vi "Анализ выхода за границы мишени (SubVI).vi"(5 "Ref мишени":refnum<vi>, 8 "Ref XY лазера":refnum<vi>, 9 "error in":errorcluster, 10 "Шаг перехода":string) -> (12 "Шаг перехода вых":string, 14 "вышел за рамки сверху":bool, 15 "вышел за рамки снизу":bool, 16 "вышел за рамки слева":bool, 17 "вышел за рамки справа":bool, 19 "error out":errorcluster)   [LabVIEW 2013]
doc: "Анализ нахождения лазера внутри мишени..."
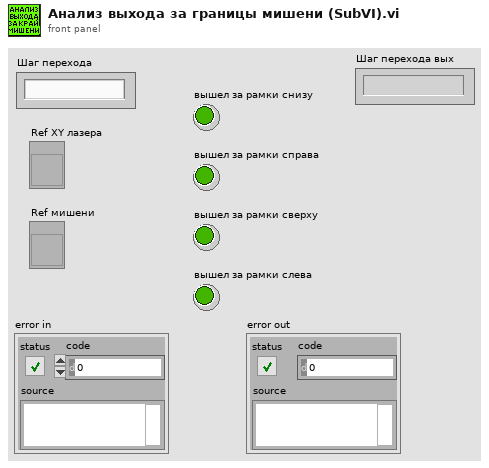
[diagram p1: front panel]
types:
  T1 = typedef "LVPositionTypeDef.ctl" = cluster{"Left":i32, "Top":i32}
  T2 = typedef "LVBoundsTypeDef.ctl" = cluster{"Width":u32, "Height":u32}
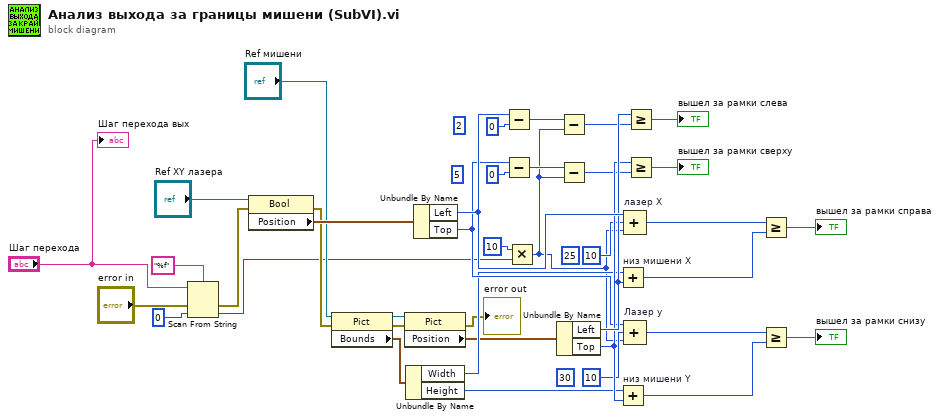
[diagram p0: block diagram]
diagram:
  (unwired) 30 ("y")
  (unwired) 25 ("y")
  (unwired) 5 ("y")
  (unwired) 2 ("y")
  n1 = Scan From String(format string="%f", input string="Шаг перехода", error in="error in", default 1=u8 0 ("element")) -> (error out=w8:errorcluster, output 1=w13:u8)  [unwired: 1 in, 2 out]
  n2 = property on="Property Node" class="Bool"(reference="Ref XY лазера", error in=w8) -> (error out=w16:errorcluster, "Position"=w20:T1)  [unwired: 1 out]
  n3 = property on="Property Node" class="Pict"(reference="Ref мишени", error in=w16) -> (reference out=w7:refnum<vi>, error out=w15:errorcluster, "Bounds"=w23:T2)
  n4 = property on="Property Node" class="Pict"(reference=w7, error in=w15) -> (error out=→"error out":errorcluster, "Position"=w19:T1)  [unwired: 1 out]
  n5 = Unbundle By Name(w23) -> ("Width"=w25:u32, "Height"=w24:u32)
  n6 = Unbundle By Name(w20) -> ("Left"=w36:i32, "Top"=w31:i32)
  n7 = Subtract(x=w36, y=0) -> (x-y=w5:i32)
  n8 = Subtract(x=w31, y=0) -> (x-y=w3:i32)
  n9 = Multiply(x=u8 10 ("element"), y=w13) -> (x*y=w2:u8)
  n10 = Unbundle By Name(w19) -> ("Left"=w33:i32, "Top"=w32:i32)
  n11 = Subtract(x=w5, y=w2) -> (x-y=w4:i32)
  n12 = Subtract(x=w3, y=w2) -> (x-y=w1:i32)
  n13 = Add "низ мишени X"(x=w25, y=w33) -> (x+y=w26:u32)
  n14 = Add "низ мишени Y"(x=w24, y=w32) -> (x+y=w39:u32)
  n15 = Compound Arithmetic op=ADD "лазер Х"(w36, 10 ("y"), w2) -> (w34:i32)
  n16 = Compound Arithmetic op=ADD "Лазер у"(w31, 10 ("y"), w2) -> (w38:i32)
  n17 = Greater Or Equal?(x=w33, y=w4) -> (x >= y?=→"вышел за рамки слева":bool)
  n18 = Greater Or Equal?(x=w32, y=w1) -> (x >= y?=→"вышел за рамки сверху":bool)
  n19 = Greater Or Equal?(x=w34, y=w26) -> (x >= y?=→"вышел за рамки справа":bool)
  n20 = Greater Or Equal?(x=w38, y=w39) -> (x >= y?=→"вышел за рамки снизу":bool)
  "Шаг перехода вых" <- "Шаг перехода"
